vi "Unregister From User Event.vi"(8 "Error In":errorcluster, 11 "User Event Registration Reference":T1) -> (0 "Error Out":errorcluster)   [LabVIEW 2023, in "QSM - Alarms.lvlib"]
doc: "This VI unregisters from the user event for the Queued Message Handler template."
uses:
  QSM - Alarms.lvlib
  Controls/User Event Registration Reference.ctl
  Controls/User Event Reference.ctl
  Controls/User Event Type.ctl
  Controls/Event Handler Message.ctl
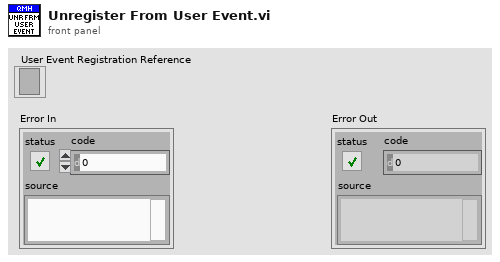
[diagram p1: front panel]
types:
  T1 = typedef "QSM - Alarms.lvlib/User Event Registration Reference.ctl" = refnum<event-registration>
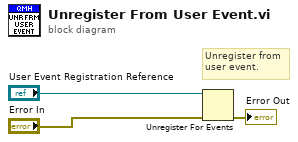
[diagram p0: block diagram]
diagram:
  # "Unregister from\nuser event."
  n1 = Unregister For Events(event registration refnum="User Event Registration Reference", error in="Error In") -> (error out=→"Error Out":errorcluster)
